vi "Update Elevator State.vi"(8 "error in (no error)":errorcluster, 10 "State in":T1, 11 "Elevator Inputs":T2) -> (0 "error out":errorcluster, 1 "Notify when settled?":bool, 2 "State out":T1, 3 "Elevator Inputs":T2)   [LabVIEW 2014]
uses:
  Elevator States.ctl
  Elevator Input Data.ctl
  Robot Global Data.vi
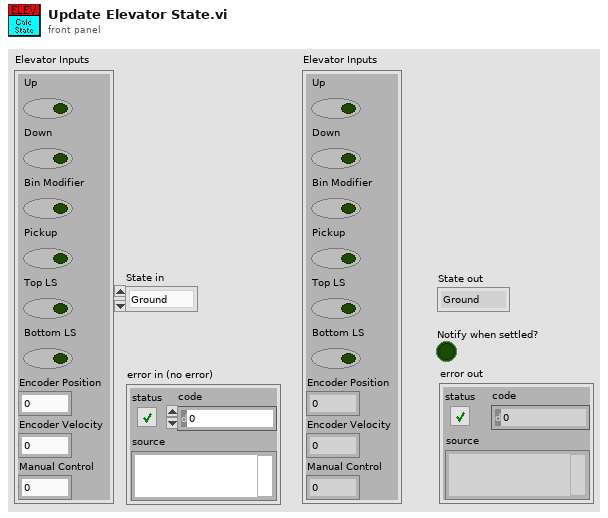
[diagram p1: front panel]
types:
  T1 = typedef "Elevator States.ctl" = enum16{"Ground", "Tote 1", "Tote 2", "Tote 3", "Tote 4", "Tote 5", "Tote 6"}
  T2 = typedef "Elevator Input Data.ctl" = cluster{"Up":bool, "Down":bool, "Bin Modifier":bool, "Pickup":bool, "Top LS":bool, "Bottom LS":bool, "Encoder Position":dbl, "Encoder Velocity":dbl, "Manual Control":dbl}
  T3 = typedef "WPI_DriverStationRobotMode2.ctl" = enum16{"Autonomous Disabled", "Autonomous Enabled", "Teleop Disabled", "Teleop Enabled", "Disconnected", "Finish", "Test Disabled", "Test Enabled", "Emergency Stopped"}
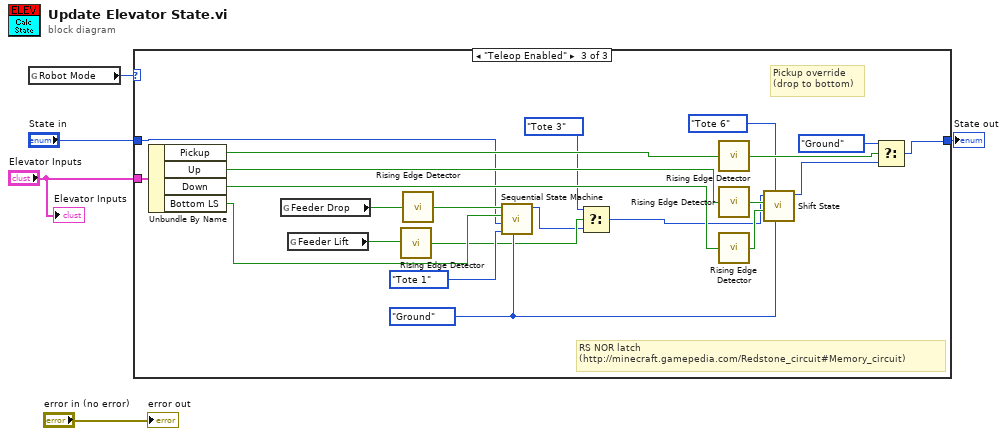
[diagram p0: block diagram]
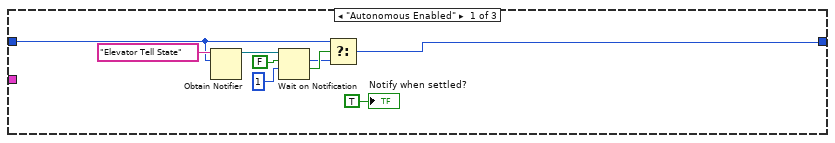
[diagram p2: hidden frame]
diagram:
  n1 = global read "Robot Global Data.vi" "Robot Mode"() -> (w4:T3)
  n2 = case shown="\"Teleop Enabled\"" w4 {
    tunnel: "State in" -> [w9 w15 w22]
    tunnel: [w8 w15 w24] -> w3
    tunnel: "Elevator Inputs" -> [_ _ w30]
    frame "Autonomous Enabled" {
      n3 = Obtain Notifier(name (unnamed)="Elevator Tell State", notification data type=w9) -> (notifier out=w13:refnum<notifier>)  [unwired: 2 in, 2 out]
      n4 = Wait on Notification(notifier=w13, ignore previous (F)=FALSE, timeout in ms (-1)=1) -> (notification=w10:T1, timed out?=w11:bool)  [unwired: 1 in, 2 out]
      n5 = Select(t=w9, s=w11, f=w10) -> (s? t:f=w8:T1)
      "Notify when settled?" <- TRUE ("Notify when settled?")
    }
    frame Default {
    }
    frame "Teleop Enabled" {
      w21 = Elevator_States."Ground" ("upper limit")
      # "RS NOR latch\n(http://minecraft.gamepedia.com/Redstone_circuit#Memory_circuit)"
      # "Pickup override\n(drop to bottom)"
      n6 = Unbundle By Name(w30) -> ("Pickup"=w33:bool, "Up"=w32:bool, "Down"=w31:bool, "Bottom LS"=w23:bool)
      n7 = global read "Robot Global Data.vi" "Feeder Drop"() -> (w27:bool)
      n8 = global read "Robot Global Data.vi" "Feeder Lift"() -> (w26:bool)
      n9 = call "Rising Edge Detector.vi"("Input"=w26) -> ("Rising edge?"=w19:bool)
      n10 = call "Rising Edge Detector.vi"("Input"=w27) -> ("Rising edge?"=w25:bool)
      n11 = call "Sequential State Machine.vi"("Base State"=w21, "Change State"=Elevator_States."Tote 1" ("upper limit"), "Old State"=w22, "Change Condition"=w23, "Button Press"=w25) -> ("Out State"=w18:i32)  [unwired: 6 in]
      n12 = Select(t=Elevator_States."Tote 3" ("upper limit"), s=w19, f=w18) -> (s? t:f=w17:i32)
      n13 = call "Rising Edge Detector.vi"("Input"=w33) -> ("Rising edge?"=w37:bool)
      n14 = call "Rising Edge Detector.vi"("Input"=w32) -> ("Rising edge?"=w34:bool)
      n15 = call "Rising Edge Detector.vi"("Input"=w31) -> ("Rising edge?"=w35:bool)
      n16 = call "Shift State.vi"("Lower bound"=w21, "Upper bound"=Elevator_States."Tote 6" ("upper limit"), "Decrement"=w35, "Increment"=w34, "State in"=w17) -> ("State out"=w28:i32)  [unwired: 6 in]
      n17 = Select(t=Elevator_States."Ground" ("upper limit"), s=w37, f=w28) -> (s? t:f=w24:i32)
    }
  }
  "State out" <- w3
  "error out" <- "error in (no error)"
  "Elevator Inputs" <- "Elevator Inputs"
